vi "Get Name.vi"(11 "CD Template":refnum<class "NIVS_Inline HW Interface (Inline-Async).lvclass">) -> (2 "String":string)   [LabVIEW 2019, in "NIVS_Inline HW Interface (Inline-Async).lvclass"]
uses:
  NIVS_Inline HW Interface (Inline-Async).lvclass
  NIVS_Consolidated_CDW_MetaDataObj/Execution Mode.ctl
  NIVS_Consolidated_CDW_MetaDataObj/NIVS_Consolidated_CDW_MetaDataObj.lvclass
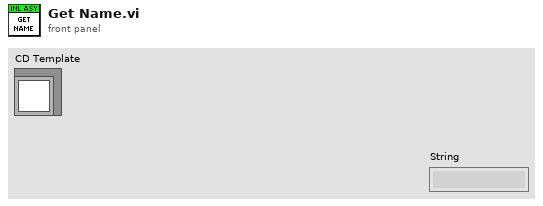
[diagram p1: front panel]
types:
  T1 = typedef "NIVS_Consolidated_CDW_MetaDataObj.lvclass/Execution Mode.ctl" = enum16{"Asynchronous", "Inline HW Interface", "Inline Model Interface", "Inline Timing and Sync", "Asynchronous Timing and Sync"}
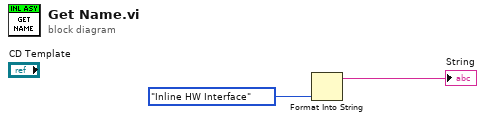
[diagram p0: block diagram]
diagram:
  n1 = Format Into String(Execution_Mode."Inline HW Interface" ("CD Execution Mode")) -> (resulting string=→"String":string)  [unwired: 3 in, 1 out]
